vi "Vision Processing (4).vi"(4 "error in (no error)":errorcluster, 5 "Camera Type":enum16{"206", "1011"}(ring)=enum."1011", 6 "Camera Name":string="Camera") -> ()   [LabVIEW 2012]
uses:
  Robot Global Data.vi
  <vilib>/vision/NI_Vision_Development_Module.lvlib
panel:
  in  "View":bool=TRUE
  out "Target Info":T1(array[cluster])
  in  "Area Size Limit %":dbl=0.5
  in  "Particle Count Limit":i32=8
  in  "Score Limits":T2={"Rect Coverage"=60.0, "X Edge Strength"=40.0, "Y Edge Strength"=60.0, "Center"=75.0, "Outer"=75.0}
  in  "Processing":enum32{"Color", "Monochrome"}(tab)
  out "Value":cluster{i32, i32}
  out "Saturation":cluster{i32, i32}
  out "Hue":cluster{i32, i32}
  in  "Luminance":i32=255
  in  "Saturation":i32=255
  in  "Hue":i32(knob)=65 scale=0.0..255.0
  in  "Margins":cluster{"Hue":i32, "Sat":i32, "Val":i32}={"Hue"=33, "Sat"=53, "Val"=9} {"Sat" scale=0.0..80.0; "Val" scale=0.0..80.0; "Hue" scale=0.0..80.0}
  in  "Range":cluster{"Lower value":sgl, "Upper value":sgl}={"Lower value"=150.0, "Upper value"=255.0} {"Lower value" scale=0.0..255.0; "Upper value" scale=0.0..255.0}
  in  "View":bool=TRUE
  out "Processed Image":T3(plugin-control)
  out "Original Image":T3(plugin-control)
  # "Instructions:\nProcessing the reflective tape that is illuminated by a ring light can be based\non color or light intensity.\nParticles within the image are scored by rectangle coverage, aspect ratio, and\nfor being hollow with a bold edge. A particle is considered a target if all scores\nare above the score limits. Particles can be annotated -- surrounded by\na rectangle and scores drawn to the left .\nTo control the number of particles being scored, use the count limit and the size\nlimit."
  # "To debug, Enable using the View button.\nFor color processing, you can click in the image to select the color for processing."
  # "Enable by clicking the View button.\nGreen scores are above the limit, orange are below. Inner/outer rect\nindicates all passed."
  # "Lower/Upper"
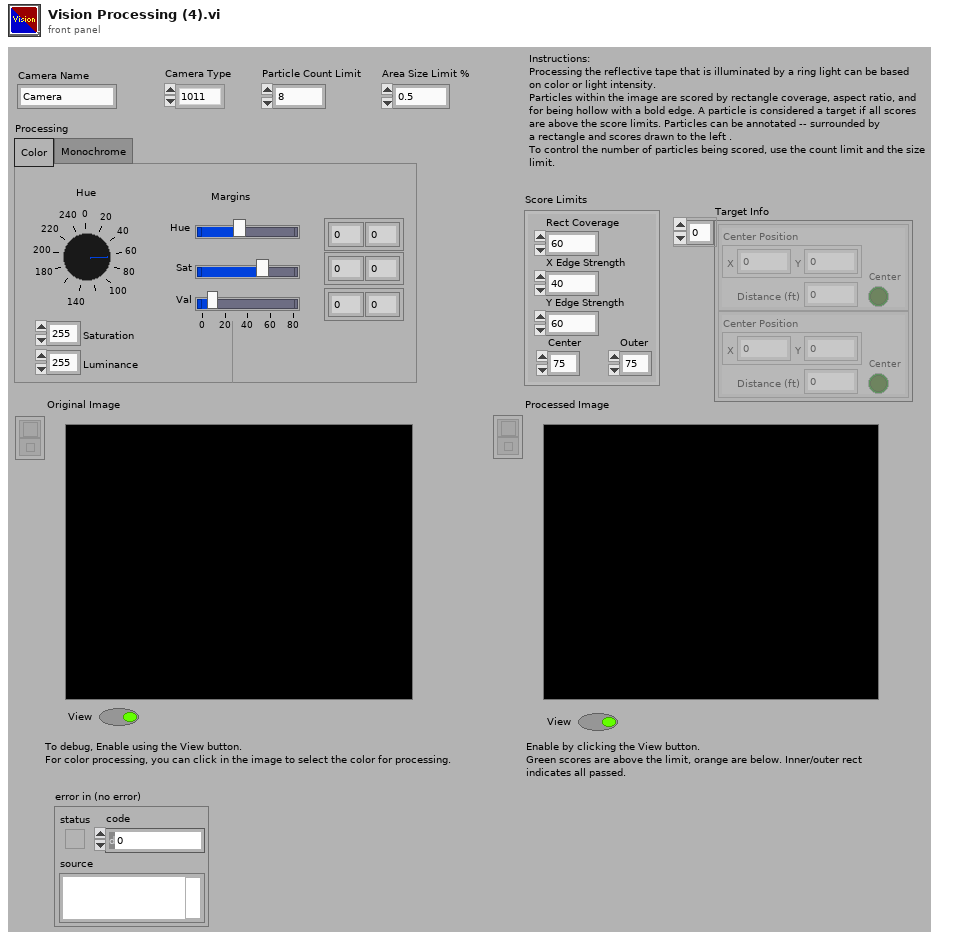
[diagram p1: front panel]
types:
  T1 = cluster{"Center Position":cluster{"X":dbl, "Y":dbl}, "Distance (ft)":dbl, "Center":bool}[]
  T2 = cluster{"Rect Coverage":dbl, "X Edge Strength":dbl, "Y Edge Strength":dbl, "Center":dbl, "Outer":dbl}
  T3 = typedef "IMAQ Image.ctl" = refnum<image>
  T4 = typedef "Image Type" = u32
  T5 = typedef "WPI_CameraDevRef.ctl" = cluster{"Camera Address":string, "CameraStatus":errorcluster, "Acquire Image Notifier":refnum<notifier>}
  T6 = cluster{"Position":cluster{"X":dbl, "Y":dbl}, "Distance (ft)":dbl, "Center":bool}[]
  T7 = typedef "WPI_CameraImageSize.ctl" = enum16{"640x480", "320x240", "160x120"}
  T8 = cluster{cluster{"Left":dbl, "Top":dbl, "Right":dbl, "Bottom":dbl}, "Scores":dbl[], cluster{"Long":dbl, "Short":dbl}}[]
  T9 = cluster{"Target Center (-1 to 1)":cluster{"X":dbl, "Y":dbl}, "Distance (ft)":dbl, "Center Target":bool}
  T10 = cluster{"Target Center (-1 to 1)":cluster{"X":dbl, "Y":dbl}, "Distance (ft)":dbl, "Center Target":bool}[]
  T11 = cluster{"Left":dbl, "Top":dbl, "Right":dbl, "Bottom":dbl}
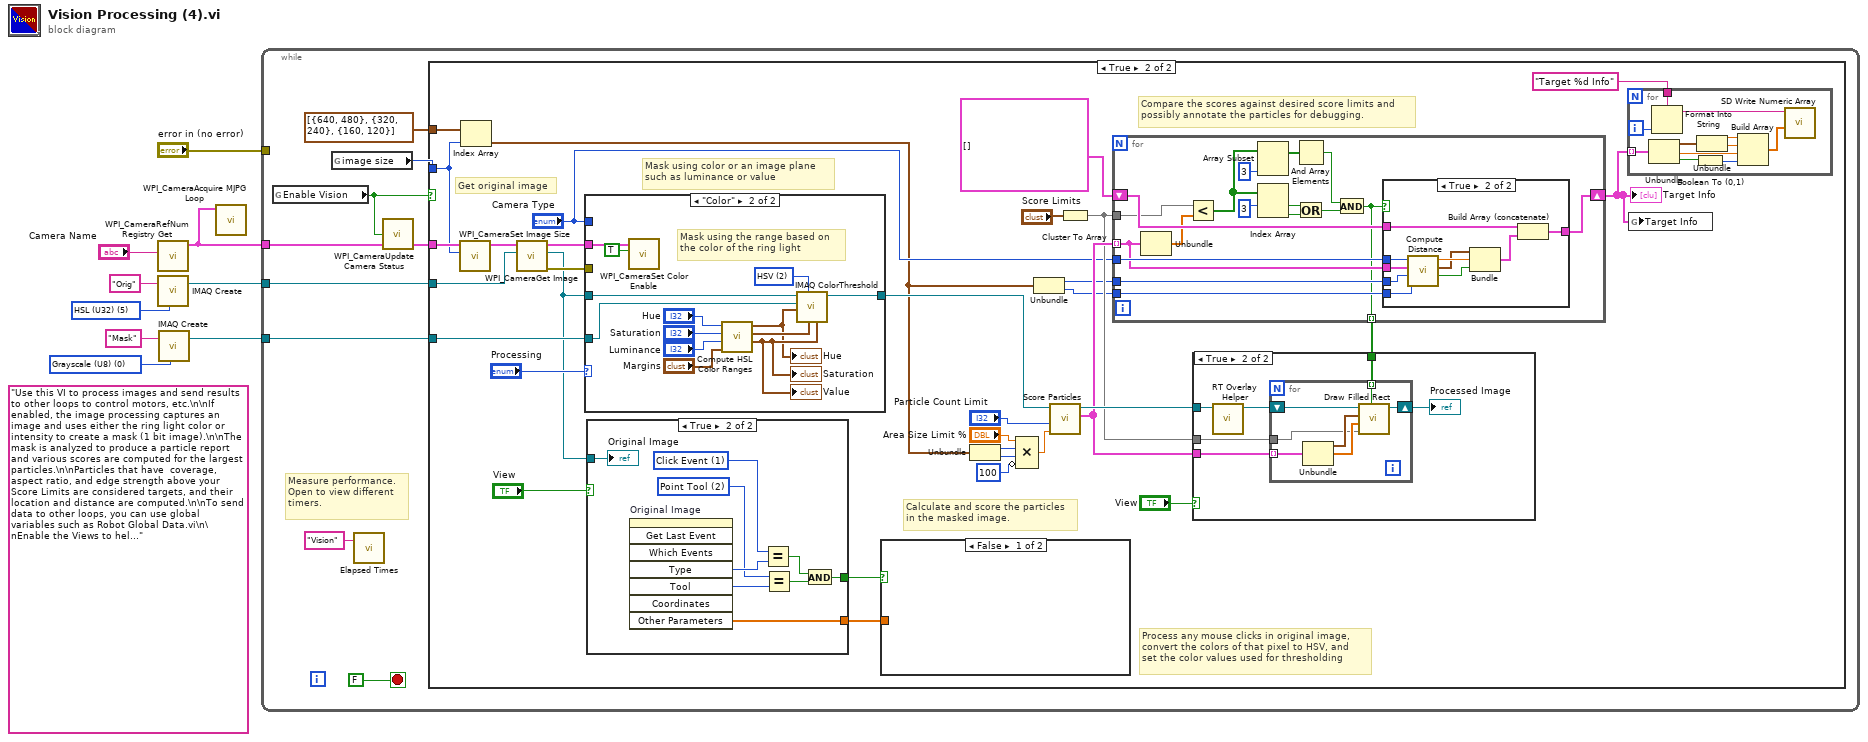
[diagram p0: block diagram]
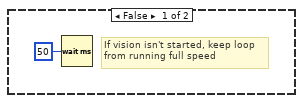
[diagram p2: hidden frame]
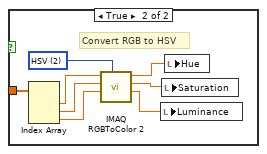
[diagram p3: hidden frame]
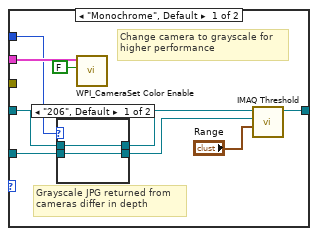
[diagram p4: hidden frame]
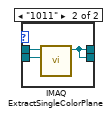
[diagram p5: hidden frame]
diagram:
  w3 = T4 0 items=["Grayscale (U8)", "Grayscale (I16)", "Grayscale (SGL)", "Complex (CSG)", "RGB (U32)", "HSL (U32)", "RGB (U64)", "Grayscale (U16)"] ("Image Type")
  (unwired) "Use this VI to process images and send results to other loops to control motors, etc.\n\nIf enabled, the image processing captures an image and uses either the ring light color or intensity to create a mask (1 bit image).\n\nThe mask is analyzed to produce a particle report and various scores are computed for the largest particles.\n\nParticles that have  coverage, aspect ratio, and edge strength above your Score Limits are considered targets, and their location and distance are computed.\n\nTo send data to other loops, you can use global variables such as Robot Global Data.vi\n\nEnable the Views to help debug color settings. Disable the View to speed up processing."
  w8 = T4 5 items=["Grayscale (U8)", "Grayscale (I16)", "Grayscale (SGL)", "Complex (CSG)", "RGB (U32)", "HSL (U32)", "RGB (U64)", "Grayscale (U16)"] ("Image Type")
  n1 = call <vilib>:"WPI_CameraRefNum Registry Get.vi"("refnum name"="Camera Name") -> ("CameraDevRef"=w5:T5)  [unwired: 9 in, 1 out]
  n2 = call "IMAQ Create"("Image Name"="Orig", "Image Type"=w8) -> ("New Image"=w7:T3)  [unwired: 2 in, 2 out]
  n3 = call "IMAQ Create"("Image Name"="Mask", "Image Type"=w3) -> ("New Image"=w1:T3)  [unwired: 2 in, 2 out]
  n4 = call <vilib>:"WPI_CameraAcquire MJPG Loop.vi"("CameraDevRef"=w5) -> ()  [unwired: 11 in]
  n5 = while {
    tunnel: w7 -> [w17]
    tunnel: w5 -> [w16]
    tunnel: "error in (no error)" -> [_]
    tunnel: w1 -> [w11]
    stop <- FALSE stop-if-true
    # "Measure performance.\nOpen to view different\ntimers."
    n6 = global read "Robot Global Data.vi" "Enable Vision"() -> (w14:bool)
    n7 = global read "Robot Global Data.vi" "image size"() -> (w12:T7)
    n8 = call "Elapsed Times.vi"("Call Name"="Vision") -> ()  [unwired: 2 in, 1 out]
    n9 = call <vilib>:"WPI_CameraUpdate Camera Status.vi"("CameraDevRef In"=w16, "Enable Vision"=w14) -> ("CameraDevRef Out"=w15:T5)  [unwired: 3 in]
    n10 = case shown="True" w14 {
      tunnel: w17 -> [_ w45]
      tunnel: w15 -> [_ w41]
      tunnel: w12 -> [_ w36]
      tunnel: w11 -> [_ w32]
      tunnel: cluster{i32, i32}[] [{640, 480}, {320, 240}, {160, 120}] -> [_ w35]
      frame False {
        # "If vision isn't started, keep loop\nfrom running full speed"
        n11 = Wait (ms)(milliseconds to wait=u32 50) -> ()  [unwired: 1 out]
      }
      frame True {
        # "Compare the scores against desired score limits and\npossibly annotate the particles for debugging."
        # "Process any mouse clicks in original image,\nconvert the colors of that pixel to HSV, and\nset the color values used for thresholding"
        # "Calculate and score the particles\nin the masked image."
        # "Mask using color or an image plane\nsuch as luminance or value"
        # "Get original image"
        n12 = call <vilib>:"WPI_CameraSet Image Size.vi"("Image Size"=w36, "CameraDevRef"=w41) -> ("CameraDevRef Out"=w42:T5)  [unwired: 8 in, 1 out]
        n13 = Index Array(array=w35, index=w36) -> (element=w21:cluster{i32, i32})
        n14 = call <vilib>:"WPI_CameraGet Image.vi"("Image"=w45, "CameraDevRef"=w42) -> ("error out"=w43:errorcluster, "Image Out"=w31:T3, "CameraDevRef Out"=w44:T5)  [unwired: 7 in]
        n15 = case shown="\"Color\"" "Processing" {
          tunnel: w31 -> [w76 w98]
          tunnel: [w79 w97] -> w39
          tunnel: w44 -> [w77 w90]
          tunnel: w43 -> [_ _]
          tunnel: w32 -> [w75 w88]
          tunnel: "Camera Type" -> [w74 _]
          frame "Monochrome", Default {
            # "Grayscale JPG returned from\ncameras differ in depth"
            # "Change camera to grayscale for\nhigher performance"
            n16 = case shown="\"206\", Default" w74 {
              tunnel: w76 -> [w82 w85]
              tunnel: w75 -> [w81 w84]
              tunnel: [w82 w83] -> w73
              tunnel: [w81 w83] -> w72
              frame "206", Default {
              }
              frame "1011" {
                n17 = call "IMAQ ExtractSingleColorPlane"("Image Dst"=w84, "Image Src"=w85) -> ("Image Dst Out"=w83:T3)  [unwired: 8 in, 1 out]
              }
            }
            n18 = call <vilib>:"WPI_CameraSet Color Enable.vi"("Color Enabled"=FALSE, "CameraDevRef"=w77) -> ()  [unwired: 8 in, 2 out]
            n19 = call "IMAQ Threshold"("Range"="Range", "Image Dst"=w72, "Image Src"=w73) -> ("Image Dst Out"=w79:T3)  [unwired: 3 in, 5 out]
          }
          frame "Color" {
            w96 = u16 2 items=["RGB", "HSL", "HSV", "HSI"] ("Color Mode")
            # "Mask using the range based on\nthe color of the ring light"
            n20 = call <vilib>:"WPI_CameraSet Color Enable.vi"("Color Enabled"=TRUE, "CameraDevRef"=w90) -> ()  [unwired: 8 in, 2 out]
            n21 = call "Compute HSL Color Ranges.vi"("Margins"="Margins", "Luminance"="Luminance", "Saturation"="Saturation", "Hue"="Hue") -> ("Lum Range"=w87:cluster{i32, i32}, "Sat Range"=w95:cluster{i32, i32}, "Hue Range"=w86:cluster{i32, i32})  [unwired: 5 in]
            "Hue" <- w86
            "Saturation" <- w87
            "Value" <- w87
            n22 = call "IMAQ ColorThreshold"("Blue or Luma or Val or Inten Range"=w87, "Green or Sat Range"=w95, "Color Mode"=w96, "Red or Hue Range"=w86, "Image Dst"=w88, "Image Src"=w98) -> ("Image Dst Out"=w97:T3)  [unwired: 4 in, 1 out]
          }
        }
        n23 = case shown="True" "View" {
          tunnel: w31 -> [_ w120]
          tunnel: [_ w115] -> w38
          tunnel: [_ w112] -> w37
          frame False {
          }
          frame True {
            w113 = 2 items=["None", "Selection Tool", "Point Tool", "Line Tool", "Rectangle Tool", "Oval Tool", "Polygon Tool", "ClosedFreehandTool", "Annulus Tool", "Rotated Rectangle Tool", "Zoom Tool", "Pan Tool", "Polyline Tool", "Freehand Tool"] ("Tool")
            w114 = 1 items=["No Event"=0, "Click Event"=1, "Draw Event"=2, "Size Event"=4, "Scroll Event"=5, "Double Click Event"=8] ("Type")
            n24 = invoke on="Original Image" class="ImageControl" method="Get Last Event"() -> ("Type"=w116:i32, "Tool"=w119:i32, "Other Parameters"=w112:sgl[])  [unwired: 8 in, 5 out]
            n25 = Equal?(x=w114, y=w116) -> (x = y?=w117:bool)
            n26 = Equal?(x=w113, y=w119) -> (x = y?=w118:bool)
            n27 = And(x=w117, y=w118) -> (x .and. y?=w115:bool)
            "Original Image" <- w120
          }
        }
        n28 = case shown="False" w38 {
          tunnel: w37 -> [_ w71]
          frame False {
          }
          frame True {
            w70 = u16 2 items=["RGB", "HSL", "HSV", "HSI", "CIE L*a*b*", "CIE XYZ"] ("Color Mode")
            # "Convert RGB to HSV"
            n29 = Index Array(array=w71) -> (element #1=w69:sgl, element #2=w67:sgl, element #3=w65:sgl)  [unwired: 3 in]
            n30 = call "IMAQ RGBToColor 2"("Color Mode"=w70, "Blue value"=w65, "Green value"=w67, "Red value"=w69) -> ("Blue or Luma or Val or Inten or Z or b*value"=w64:dbl, "Green or Sat or Y or a* value"=w66:dbl, "Red or Hue or X or L* value"=w68:dbl)  [unwired: 4 in, 1 out]
            n31 = local write "Luminance"(w64) -> ()
            n32 = local write "Saturation"(w66) -> ()
            n33 = local write "Hue"(w68) -> ()
          }
        }
        n34 = Unbundle(w21) -> (w25:i32, w24:i32)
        n35 = Compound Arithmetic op=MULTIPLY("Area Size Limit %", w25, w24, invert 100 ("length")) -> (w22:dbl)
        n36 = Unbundle(w21) -> (w34:i32, w33:i32)
        n37 = call "Score Particles.vi"("Area Size Limit"=w22, "Particle Count Limit"="Particle Count Limit", "Image Refnum in"=w39) -> ("Scored Particle Info"=w49:T8, "Image Refnum out"=w51:T3)  [unwired: 7 in]
        n38 = Cluster To Array(cluster="Score Limits") -> (array=w47:dbl[])
        n39 = for {
          shift-right: [w136] -> w20
          shift-left: T6 [] -> [w137]
          tunnel: w34 -> [w135]
          tunnel: w49 -> [w130] mode=indexing
          tunnel: w47 -> [w132]
          tunnel: "Camera Type" -> [w134]
          tunnel: w33 -> [w131]
          tunnel: [w121] -> w27 mode=indexing
          n40 = Unbundle(w130) -> ("Scores"=w133:dbl[])  [unwired: 2 out]
          n41 = Less?(x=w132, y=w133) -> (x < y?=w122:bool[])
          n42 = Array Subset(array=w122, length=3) -> (w124:bool[])  [unwired: 1 in]
          n43 = Index Array(array=w122, index #1=3 ("length")) -> (element #1=w126:bool, element #2=w127:bool)  [unwired: 1 in]
          n44 = And Array Elements(Boolean array=w124) -> (logical AND=w129:bool)
          n45 = Or(x=w126, y=w127) -> (x .or. y?=w128:bool)
          n46 = And(x=w129, y=w128) -> (x .and. y?=w121:bool)
          n47 = case shown="True" w121 {
            tunnel: w137 -> [w138 w148]
            tunnel: [w138 w147] -> w136
            tunnel: w135 -> [_ w145]
            tunnel: w134 -> [_ w143]
            tunnel: w131 -> [_ w142]
            tunnel: w130 -> [_ w140]
            frame False {
            }
            frame True {
              n48 = call "Compute Distance.vi"("Y Image Resolution"=w142, "X Image Resolution"=w145, "Particle Scores"=w140, "Camera Type"=w143) -> ("Center Target"=w139:bool, "Target Center (-1 to 1)"=w141:cluster{"X":dbl, "Y":dbl}, "Distance (ft)"=w144:dbl)  [unwired: 5 in]
              n49 = Bundle("Target Center (-1 to 1)"=w141, "Distance (ft)"=w144, "Center Target"=w139) -> (w146:T9)  [unwired: 1 in]
              n50 = Build Array (concatenate)(w148, w146) -> (w147:T10)
            }
          }
        }
        "Target Info" <- w20
        n51 = case shown="True" "View" {
          tunnel: w51 -> [_ w101]
          tunnel: w49 -> [_ w103]
          tunnel: w47 -> [_ w102]
          tunnel: w27 -> [_ w99]
          frame False {
          }
          frame True {
            n52 = call "RT Overlay Helper.vi"("Refnum in"=w101) -> ("Refnum out"=w104:T3)  [unwired: 10 in]
            n53 = for {
              shift-right: [w110] -> w100
              shift-left: w104 -> [w111]
              tunnel: w103 -> [w107] mode=indexing
              tunnel: w102 -> [w106]
              tunnel: w99 -> [w105] mode=indexing
              n54 = Unbundle(w107) -> (w108:T11, "Scores"=w109:dbl[])  [unwired: 1 out]
              n55 = call "Draw Filled Rect.vi"("Limit Passed"=w105, "Limits"=w106, "Scores"=w109, "Bounding Box"=w108, "image in"=w111) -> ("image out"=w110:T3)  [unwired: 6 in]
            }
            "Processed Image" <- w100
          }
        }
        n56 = for {
          tunnel: w20 -> [w63] mode=indexing
          tunnel: "Target %d Info" ("Name") -> [w62]
          i -> [w59]
          n57 = Unbundle(w63) -> ("Position"=w60:cluster{"X":dbl, "Y":dbl}, "Distance (ft)"=w55:dbl, "Center"=w58:bool)
          n58 = Format Into String(format string=w62, w59) -> (resulting string=w61:string)  [unwired: 2 in, 1 out]
          n59 = Boolean To (0,1)(Boolean=w58) -> (0, 1=w54:i16)
          n60 = Unbundle(w60) -> ("X"=w57:dbl, "Y"=w56:dbl)
          n61 = Build Array(w57, w56, w55, w54) -> (w53:dbl[])
          n62 = call <vilib>:"SD Write Numeric Array.vi"("Numeric Array"=w53, "Name"=w61) -> ()  [unwired: 8 in, 2 out]
        }
        n63 = global write "Robot Global Data.vi" "Target Info"(w20) -> ()
      }
    }
  }
